vi "Global_CMD_ACT_Data In.vi"() -> ()   [LabVIEW 2023, in "Pivot FX_ACT.lvlib"]
uses:
  Pivot FX_ACT.lvlib
  Cluster_CMD_ACT_Data.ctl
  ENUM_CMD_Mode Select.ctl
  Shared Code/TypeDefs/ENUM_Pivot Arm Position Select.ctl
panel:
  in  "CMD_ACT_PivotFX_Data":T1
  # "The Names of the Data items in the Global Variable MUST describe who the Single Writer is\nFor Command Globals the Commander(CMD) represents Teleop or Autonomous or other command loop.\nThe naming convention for a Command Actuator Global is:   \n\nCMD_ACT_SubSystem_Data Name\n\nExample:\nCMD_ACT_Drive_Data\nCMD_ACT_Hopper_Eject Ball"
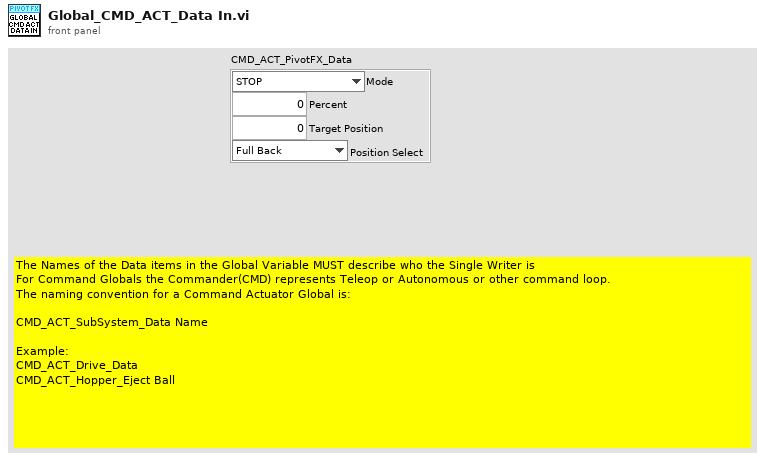
[diagram p1: front panel]
types:
  T1 = typedef "Pivot FX_ACT.lvlib/Cluster_CMD_ACT_Data.ctl" = cluster{"Mode":T2, "Percent":dbl, "Target Position":dbl, "Position Select":T3}
  T2 = typedef "Pivot FX_ACT.lvlib/ENUM_CMD_Mode Select.ctl" = enum16{"STOP", "PercentOut", "Positon Value", "Position Select"}
  T3 = typedef "ENUM_Pivot Arm Position Select.ctl" = enum16{"Full Back", "Full Forward", "Amp Score", "Pivot Arm Load", "Vertical", "Trap Score"}
diagram:
